vi "InitRestful.vi"(8 "error in (no error)":errorcluster, 11 "Device In":T2) -> (0 "error out":errorcluster, 2 "Device Out":T2={"Name"="", "BaseURL"="", "AppKey"="", "Headers"=["Content-Type:application/json"], "Timeout"=10000, "Identifier"="", "Password"="", "Comments"="", "Handle"=0, "# Handles"=0}, 3 "Refnum out":T1)   [LabVIEW 2016]
uses:
  <vilib>/httpClient/LabVIEWHTTPClient.lvlib
  <vilib>/httpClient/ClientHandle.ctl
  RWPrefCluster.vi
  Device.ctl
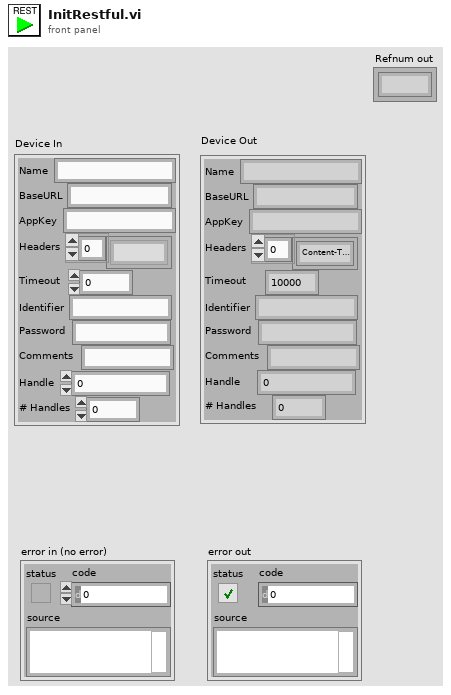
[diagram p1: front panel]
types:
  T1 = typedef "LabVIEWHTTPClient.lvlib/ClientHandle.ctl" = refnum<k1>
  T2 = typedef "Device.ctl" = cluster{"Name":string, "BaseURL":string, "AppKey":string, "Headers":string[], "Timeout":i32, "Identifier":string, "Password":string, "Comments":string, "Handle":u32, "# Handles":i32}
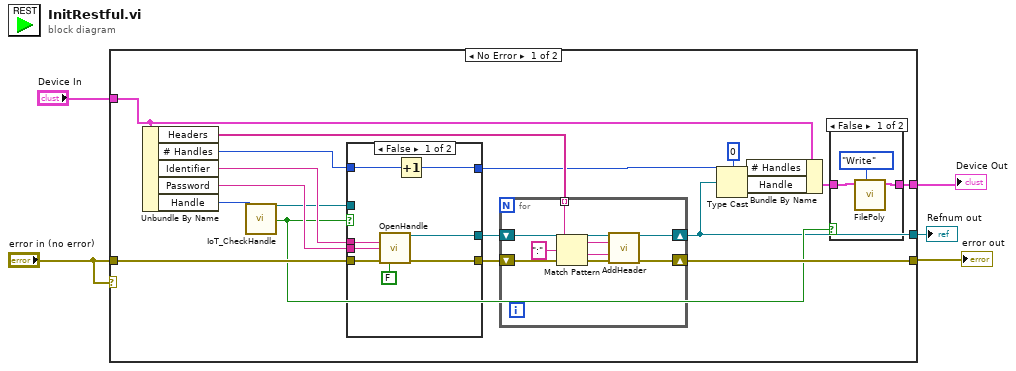
[diagram p0: block diagram]
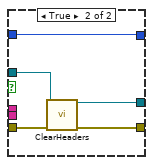
[diagram p3: hidden frame]
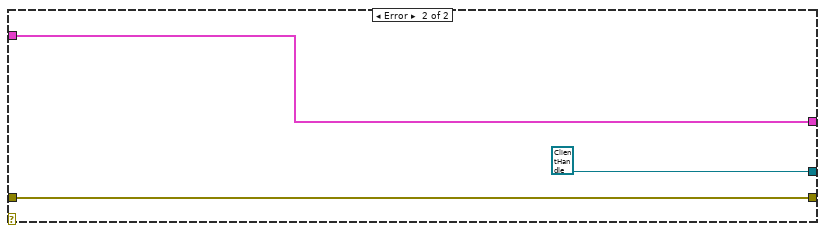
[diagram p4: hidden frame]
diagram:
  n1 = case shown="No Error" "error in (no error)" {
    tunnel: "Device In" -> [w23 w51]
    tunnel: [w22 w50] -> w4
    tunnel: "error in (no error)" -> [w21 w50]
    tunnel: [w8 w51] -> w3
    tunnel: [w6 T1 refnum ("client handle out")] -> w1
    frame No Error {
      n2 = Unbundle By Name(w23) -> ("Headers"=w17:string[], "# Handles"=w11:i32, "Identifier"=w19:string, "Password"=w20:string, "Handle"=w14:u32)
      n3 = call "IoT_CheckHandle.vi"("Handle in"=w14) -> ("Good Handle?"=w7:bool, "Refnum out"=w13:T1)  [unwired: 9 in]
      n4 = case shown="False" w7 {
        tunnel: [w35 w37] -> w18
        tunnel: [w34 w39] -> w12
        tunnel: w21 -> [w32 w38]
        tunnel: w19 -> [w31 _]
        tunnel: w20 -> [w30 _]
        tunnel: w13 -> [_ w40]
        tunnel: [w28 w36] -> w10
        tunnel: w11 -> [w29 w36]
        frame False {
          n5 = call <vilib>:"OpenHandle.vi"("username"=w31, "password"=w30, "error in (no error)"=w32, "verify server(true)"=FALSE) -> ("client handle out"=w34:T1, "error out"=w35:errorcluster)  [unwired: 10 in]
          n6 = Increment(x=w29) -> (x+1=w28:i32)
        }
        frame True {
          n7 = call "ClearHeaders.vi"("error in (no error)"=w38, "Refnum in"=w40) -> ("error out"=w37:errorcluster, "Refnum out"=w39:T1)  [unwired: 8 in]
        }
      }
      n8 = for {
        shift-right: [w47] -> w6
        shift-left: w12 -> [w48]
        shift-right: [w45] -> w22
        shift-left: w18 -> [w46]
        tunnel: w17 -> [w41] mode=indexing
        n9 = Match Pattern(string=w41, regular expression=":") -> (before substring=w43:string, after substring=w42:string)  [unwired: 1 in, 2 out]
        n10 = call <vilib>:"AddHeader.vi"("client handle"=w48, "header"=w43, "value"=w42, "error in (no error)"=w46) -> ("client handle out"=w47:T1, "error out"=w45:errorcluster)  [unwired: 10 in]
      }
      n11 = Type Cast(type=u32 0 ("y"), x=w6) -> (*(type *) &x=w15:u32)
      n12 = Bundle By Name(cluster=w23, "# Handles"=w10, "Handle"=w15) -> (w9:T2)
      n13 = case shown="False" w7 {
        tunnel: w9 -> [w25 w27]
        tunnel: [w24 w27] -> w8
        frame False {
          n14 = call-poly "FilePoly.vi"("Task"=enum16{"Read", "Write"}."Write", "Device In"=w25) -> ("Device Out"=w24:T2)  [unwired: 8 in, 1 out]
        }
        frame True {
        }
      }
    }
    frame Error {
    }
  }
  "Device Out" <- w3
  "error out" <- w4
  "Refnum out" <- w1
